vi "TDC_configureSelftest.vi"(0 "Channel Mask":i32, 5 "Period [20ns]":i32=2 min=2 max=60, 7 "Burst Size":i32=1 min=1 max=65535, 9 "Burst Distance [80 ns]":i32 min=0 max=10000, 11 "Error In":errorcluster) -> (15 "Error Out":errorcluster)   [LabVIEW 2011]
uses:
  dist/userlib/lib/tdcbase.dll
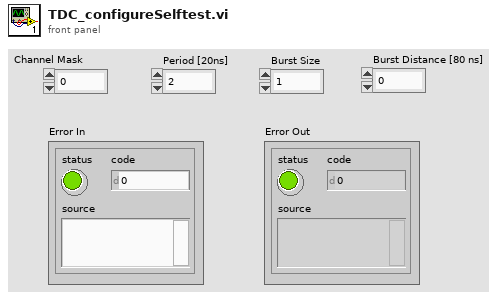
[diagram p1: front panel]
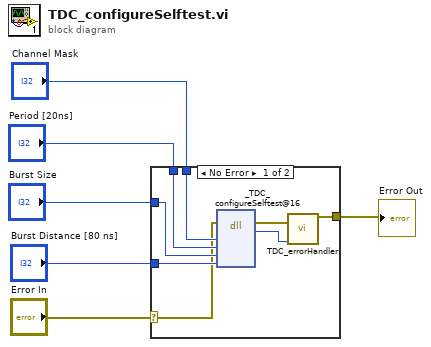
[diagram p0: block diagram]
diagram:
  n1 = case shown="No Error" "Error In" {
    selector: "Error In" -> [w10 w15]
    tunnel: [w7 w15] -> w5
    tunnel: "Channel Mask" -> [w14 _]
    tunnel: "Period [20ns]" -> [w13 _]
    tunnel: "Burst Size" -> [w12 _]
    tunnel: "Burst Distance [80 ns]" -> [w11 _]
    frame No Error {
      n2 = dll-call lib="C:/nh/projekt/spmctrl/dist/userlib/lib/tdcbase.dll" fn="_TDC_configureSelftest@16"(error in=w10, "channelMask"=w14, "period"=w13, "burstSize"=w12, "burstDist"=w11) -> (error out=w9:errorcluster, "return type"=w8:i32)  [unwired: 6 in, 1 out]
      n3 = call "TDC_errorHandler.vi"("quTAU Return Code"=w8, "Error In"=w9) -> ("Error Out"=w7:errorcluster)  [unwired: 9 in]
    }
    frame Error {
    }
  }
  "Error Out" <- w5
